vi "WILT Agilent Channels.vi"(0 "file path (dialog if empty)":path=path "C:/Users/220038920/Desktop/Project/NI-2010/Trunk/Dryer Wilt/Documentation/Agilent Channel Assignment - Wilt.ini") -> (3 "Temperature Channels":T2[](array[typedef]), 4 "Data Out Array":T1, 8 "Agilent Channels Raw":T2[](array[typedef]), 10 "Agilent Channels To Read":T2[](array[typedef]), 14 "Start Buttons":T2[](array[typedef]), 15 "Agilent Channel Water Valves":T2[](array[typedef]))   [LabVIEW 2016]
uses:
  Type Definitions/WILT Agilent Channel Definition.ctl
  Type Definitions/WILT Agilent Data Cluster.ctl
  <vilib>/Utility/file.llb/Read From Spreadsheet File (string).vi
panel:
  in  "Tab Control":enum32{"Output Data", "Extra", "Raw Data"}(tab)
  out "all rows":string[][](array[string])
  # "This is the index of all of the channel locations \nin the Agilent DBL array. Each row represents a station.\nThe station labels are below"
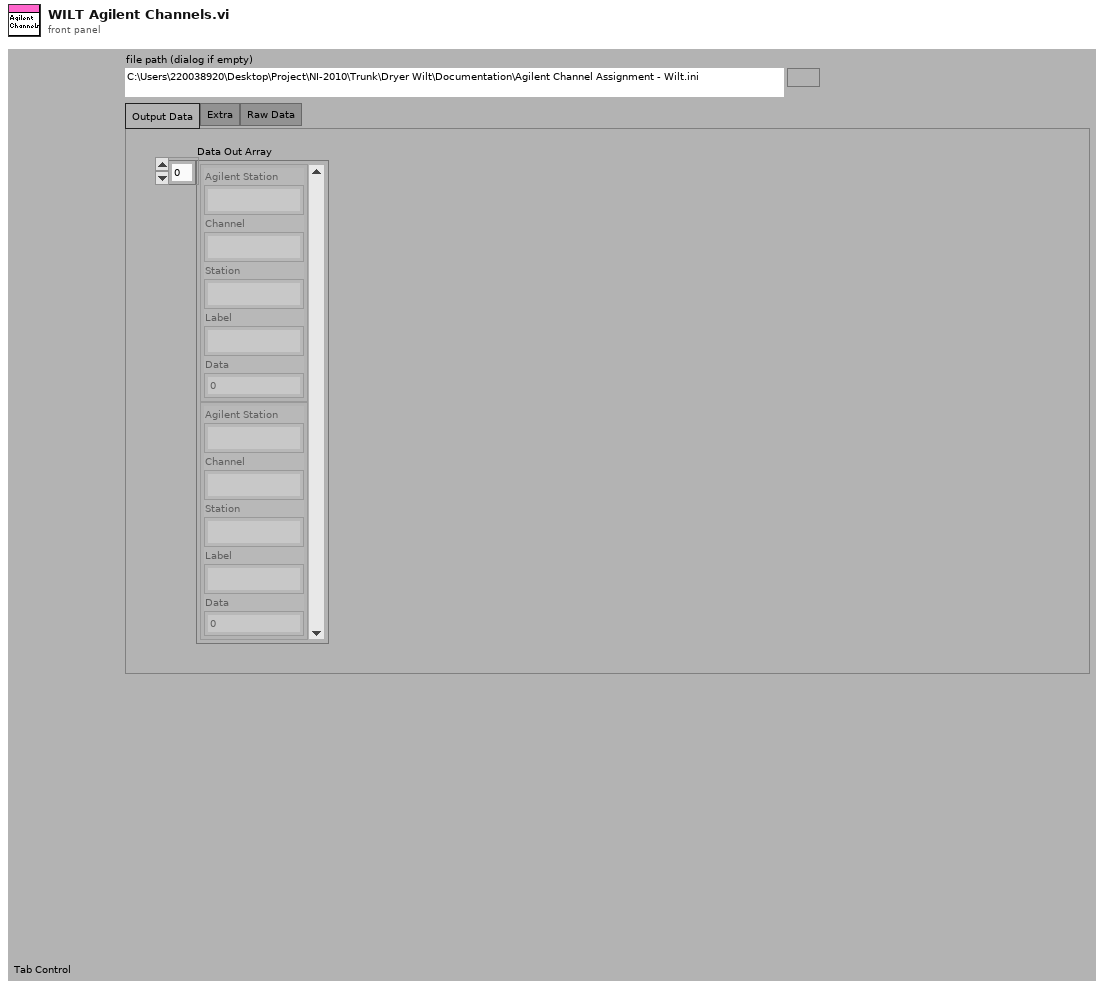
[diagram p1: front panel]
types:
  T1 = typedef "WILT Agilent Data Cluster.ctl" = T2[]
  T2 = typedef "WILT Agilent Channel Definition.ctl" = cluster{"Channel":string, "Station":string, "Label":string, "Agilent Station":string, "Data":dbl}
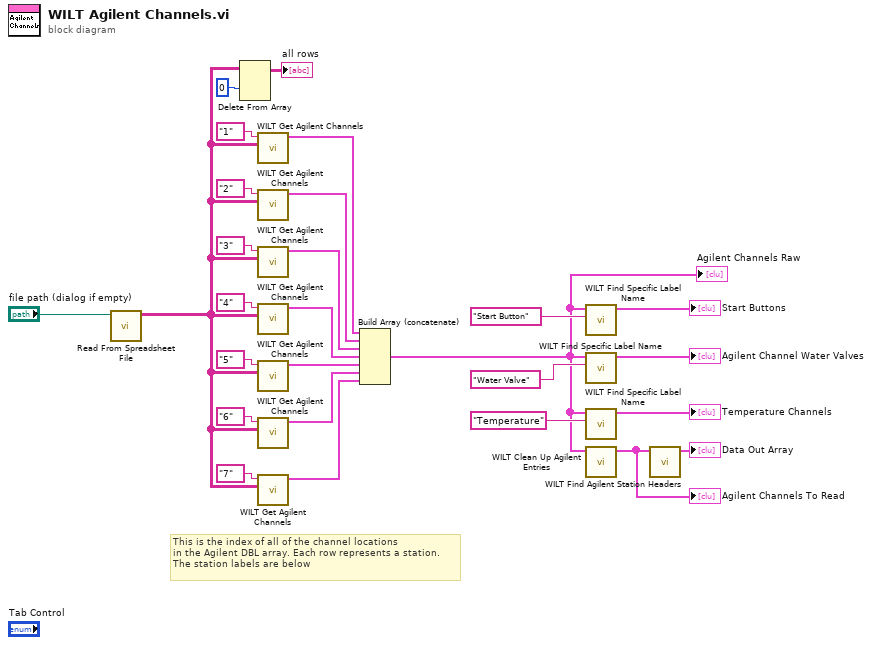
[diagram p0: block diagram]
diagram:
  # "This is the index of all of the channel locations \nin the Agilent DBL array. Each row represents a station.\nThe station labels are below"
  n1 = call-poly <vilib>:"Read From Spreadsheet File.vi"("file path (dialog if empty)"="file path (dialog if empty)") -> ("all rows"=w4:string[][])  [unwired: 6 in, 4 out]
  n2 = Delete From Array(array=w4, index (row)=0 ("disabled index (col)")) -> (array with subset deleted=→"all rows":string[][])  [unwired: 2 in, 1 out]
  n3 = call "WILT Get Agilent Channels.vi"("all rows"=w4, "Agilent Channel"="1" ("Agilent Station")) -> ("Agilent Control"=w20:T2[])  [unwired: 9 in]
  n4 = call "WILT Get Agilent Channels.vi"("all rows"=w4, "Agilent Channel"="2" ("Agilent Station")) -> ("Agilent Control"=w19:T2[])  [unwired: 9 in]
  n5 = call "WILT Get Agilent Channels.vi"("all rows"=w4, "Agilent Channel"="3" ("Agilent Station")) -> ("Agilent Control"=w18:T2[])  [unwired: 9 in]
  n6 = call "WILT Get Agilent Channels.vi"("all rows"=w4, "Agilent Channel"="4" ("Agilent Station")) -> ("Agilent Control"=w17:T2[])  [unwired: 9 in]
  n7 = call "WILT Get Agilent Channels.vi"("all rows"=w4, "Agilent Channel"="5" ("Agilent Station")) -> ("Agilent Control"=w16:T2[])  [unwired: 9 in]
  n8 = call "WILT Get Agilent Channels.vi"("all rows"=w4, "Agilent Channel"="6" ("Agilent Station")) -> ("Agilent Control"=w15:T2[])  [unwired: 9 in]
  n9 = call "WILT Get Agilent Channels.vi"("all rows"=w4, "Agilent Channel"="7" ("Agilent Station")) -> ("Agilent Control"=w2:T2[])  [unwired: 9 in]
  n10 = Build Array (concatenate)(w20, w19, w18, w17, w16, w15, w2) -> (w9:T2[])
  "Agilent Channels Raw" <- w9
  n11 = call "WILT Find Specific Label Name.vi"("Search Label Name"="Start Button" ("y"), "Agilent Channels Raw"=w9) -> ("Specific"=→"Start Buttons":T2[])  [unwired: 9 in]
  n12 = call "WILT Find Specific Label Name.vi"("Search Label Name"="Water Valve", "Agilent Channels Raw"=w9) -> ("Specific"=→"Agilent Channel Water Valves":T2[])  [unwired: 9 in]
  n13 = call "WILT Find Specific Label Name.vi"("Search Label Name"="Temperature" ("y"), "Agilent Channels Raw"=w9) -> ("Specific"=→"Temperature Channels":T2[])  [unwired: 9 in]
  n14 = call "WILT Clean Up Agilent Entries.vi"("Agilent Channels Raw"=w9) -> ("Full Agilent Array"=w8:T2[])  [unwired: 10 in]
  "Agilent Channels To Read" <- w8
  n15 = call "WILT Find Agilent Station Headers.vi"("Full Agilent Array"=w8) -> ("Data Out Array"=→"Data Out Array":T1)  [unwired: 10 in]
